vi "Instrument Update sDriverId for Spartan 6.0.vi"(8 "error in (no error)":errorcluster, 11 "Connection Refnum":T1) -> (0 "error out":errorcluster, 3 "Connection Refnum":T1)   [LabVIEW 2011]
uses:
  SI.LIB/ODBC/SQL Controls/Connection Refnum.ctl
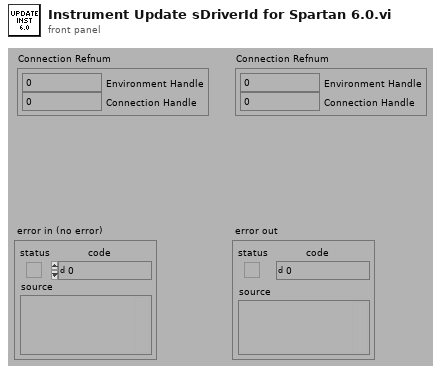
[diagram p1: front panel]
types:
  T1 = typedef "Connection Refnum.ctl" = cluster{"Environment Handle":i32, "Connection Handle":i32}
  T2 = typedef "Instrument Record.ctl" = cluster{"ixInstrument":i32, "sxInstrumentId":string, "sDriverId":string, "sDriverType":string, "sSerialNumber":string, "tLastCalibration":timestamp, "tCalibrationDue":timestamp, "sConfiguration":string}
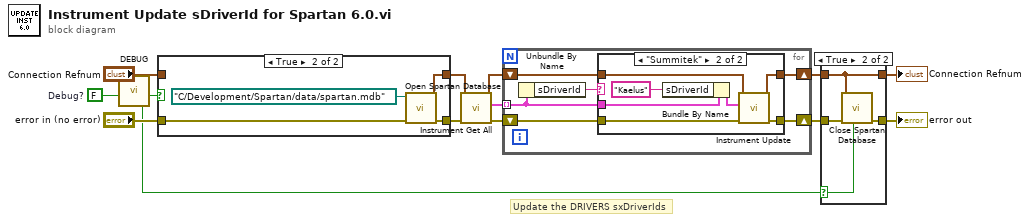
[diagram p0: block diagram]
diagram:
  w9 = FALSE  # Debug?
  # "Update the DRIVERS sxDriverIds"
  n1 = call "DEBUG.vi"("Dev DEBUG? (f)"=w9) -> ("DEBUG?"=w8:bool)  [unwired: 1 in, 5 out]
  n2 = case shown="True" w8 {
    tunnel: "Connection Refnum" -> [w15 _]
    tunnel: "error in (no error)" -> [w14 w19]
    tunnel: [w14 w18] -> w1
    tunnel: [w15 w17] -> w2
    frame False {
    }
    frame True {
      n3 = call "Open Spartan Database.vi"("error in (no error)"=w19, "DB Path (empty - use default)"=path "C:/Development/Spartan/data/spartan.mdb" ("DB Path")) -> ("error out"=w18:errorcluster, "Connection Refnum"=w17:T1)  [unwired: 1 in, 7 out]
    }
  }
  n4 = call "Instrument Get All.vi"("error in (no error)"=w1, "Connection Refnum"=w2) -> ("error out"=w7:errorcluster, "Instruments"=w3:T2[], "Connection Refnum"=w5:T1)  [unwired: 6 in, 1 out]
  n5 = for {
    shift-right: [w22] -> w4
    shift-left: w5 -> [w23]
    tunnel: w3 -> [w21] mode=indexing
    shift-right: [w24] -> w6
    shift-left: w7 -> [w25]
    n6 = Unbundle By Name(w21) -> ("sDriverId"=w20:string)
    n7 = case shown="\"Summitek\"" w20 {
      tunnel: w25 -> [w26 w34]
      tunnel: [w26 w33] -> w24
      tunnel: w23 -> [w27 w32]
      tunnel: [w27 w29] -> w22
      tunnel: w21 -> [_ w31]
      frame Default {
      }
      frame "Summitek" {
        n8 = Bundle By Name(cluster=w31, "sDriverId"="Kaelus" ("sxDriverId")) -> (w30:T2)
        n9 = call "Instrument Update.vi"("error in (no error)"=w34, "Instrument Record"=w30, "Connection Refnum"=w32) -> ("error out"=w33:errorcluster, "Connection Refnum"=w29:T1)  [unwired: 6 in, 1 out]
      }
    }
  }
  n10 = case shown="True" w8 {
    selector: w8 -> [_ w37]
    tunnel: w6 -> [w36 w40]
    tunnel: w4 -> [w35 w38]
    tunnel: [w35 w38] -> w13
    tunnel: [w36 w39] -> w12
    frame False {
    }
    frame True {
      n11 = call "Close Spartan Database.vi"("Force Close? (f)"=w37, "error in (no error)"=w40, "Connection Refnum"=w38) -> ("error out"=w39:errorcluster)  [unwired: 2 in, 6 out]
    }
  }
  "error out" <- w12
  "Connection Refnum" <- w13
